vi "synchronize.vi"(8 "error in (no error)":errorcluster, 10 "input complex waveform":cluster{"t0":dbl, "dt":dbl, "Y":cdb[]}, 11 "Modulation Parameters In":T1={"RX Parameters"={"RX Oversample Factor"=4, "RX Sample Rate"=4000000.0, "Synchronization Options"={"Synchronization Method"=enum."Fixed Offset", "Symbol Timing Recovery Method "=enum."MT Allign To Ideal Symbols", "Fixed Offset"=0.0, "Frame Detection Method"=enum."", "Correct Frequency Offset"=FALSE}, "Channel Estimation/Equalization Parameters"={"Equalization Method"=enum."", "Channel Estimate Length"=0.0, "Equalizer Length"=0.0, "Equalizer Delay"=0.0}}, "TX/RX Shared Parameters"={"Modulation Type"=enum."OOK", "Packet Length"=128, "# of Iterations"=0.0, "Pulse Shaping Parameters"={"Pulse Shaping Filter"=enum."none", "Filter Length (symbols)"=32, "Filter Parameter"=0.8, "modulation type"=enum."FSK"}, "Header/Tail Control Information"={"Training Sequence Type"=enum."", "Zero Pad Length"=0.0}}}) -> (0 "error out":errorcluster, 2 "output complex waveform":cluster{"t0":dbl, "dt":dbl, "Y":cdb[]}, 3 "Modulation Parameters Out":T1={"RX Parameters"={"RX Oversample Factor"=4, "RX Sample Rate"=4000000.0, "Synchronization Options"={"Synchronization Method"=enum."Fixed Offset", "Symbol Timing Recovery Method "=enum."MT Allign To Ideal Symbols", "Fixed Offset"=0.0, "Frame Detection Method"=enum."", "Correct Frequency Offset"=FALSE}, "Channel Estimation/Equalization Parameters"={"Equalization Method"=enum."", "Channel Estimate Length"=0.0, "Equalizer Length"=0.0, "Equalizer Delay"=0.0}}, "TX/RX Shared Parameters"={"Modulation Type"=enum."OOK", "Packet Length"=128, "# of Iterations"=0.0, "Pulse Shaping Parameters"={"Pulse Shaping Filter"=enum."none", "Filter Length (symbols)"=32, "Filter Parameter"=0.8, "modulation type"=enum."FSK"}, "Header/Tail Control Information"={"Training Sequence Type"=enum."", "Zero Pad Length"=0.0}}})   [LabVIEW 2012]
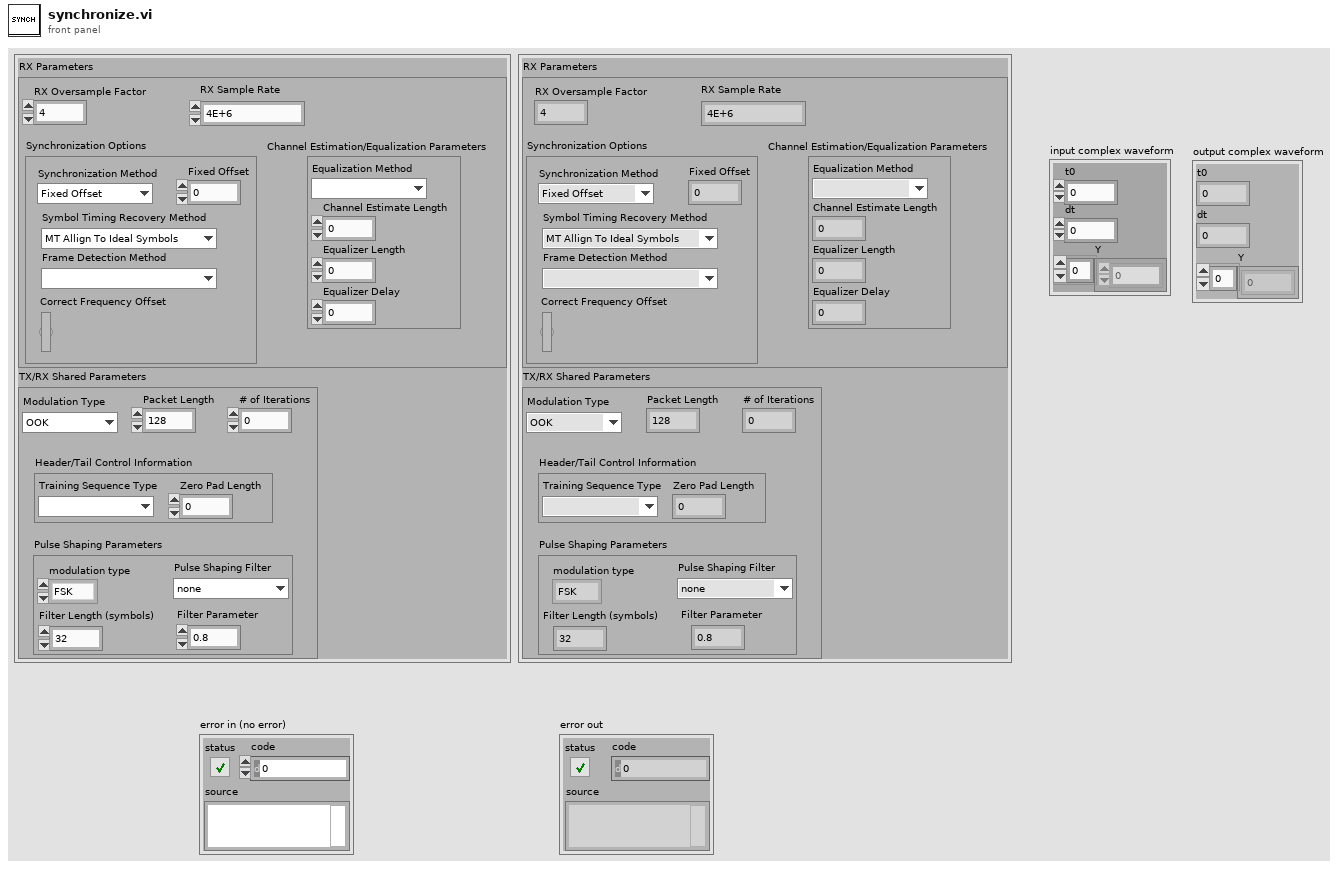
[diagram p1: front panel]
types:
  T1 = cluster{"RX Parameters":cluster{"RX Oversample Factor":i32, "RX Sample Rate":dbl, "Synchronization Options":cluster{"Synchronization Method":enum16{"Fixed Offset", "Timing Estimation", "Joint Timing and Channel Estimation"}, "Symbol Timing Recovery Method ":enum16{"MT Allign To Ideal Symbols", "Maximum Energy", "Early-Late Gate", "Gardner", "Fixed Offset"}, "Fixed Offset":dbl, "Frame Detection Method":enum16{""}, "Correct Frequency Offset":bool}, "Channel Estimation/Equalization Parameters":cluster{"Equalization Method":enum16{""}, "Channel Estimate Length":dbl, "Equalizer Length":dbl, "Equalizer Delay":dbl}}, "TX/RX Shared Parameters":cluster{"Modulation Type":enum16{"OOK", "FSK"}, "Packet Length":i32, "# of Iterations":dbl, "Pulse Shaping Parameters":cluster{"Pulse Shaping Filter":enum16{"none", "Raised Cosine", "Root Raised Cos", "Gaussian"}, "Filter Length (symbols)":i32, "Filter Parameter":dbl, "modulation type":enum16{"FSK", "PSK", "QAM", "MSK", "PAM", "ASK", "CPM"}}, "Header/Tail Control Information":cluster{"Training Sequence Type":enum16{""}, "Zero Pad Length":dbl}}}
  T2 = enum16{"Fixed Offset", "Timing Estimation", "Joint Timing and Channel Estimation"}
  T3 = cluster{"RX Parameters":cluster{"RX Oversample Factor":i32, "RX Sample Rate":dbl, "Synchronization Options":cluster{"Synchronization Method":enum16{"Fixed Offset", "Timing Estimation", "Joint Timing and Channel Estimation"}, "Symbol Timing Recovery Method ":enum16{"MT Allign To Ideal Symbols", "Maximum Energy", "Early-Late Gate", "Gardner", "Fixed Offset"}, "Fixed Offset":i32, "Frame Detection Method":enum16{""}, "Correct Frequency Offset":bool}, "Channel Estimation/Equalization Parameters":cluster{"Equalization Method":enum16{""}, "Channel Estimate Length":dbl, "Equalizer Length":dbl, "Equalizer Delay":dbl}}, "TX/RX Shared Parameters":cluster{"Modulation Type":enum16{"OOK", "FSK"}, "Packet Length":i32, "# of Iterations":dbl, "Pulse Shaping Parameters":cluster{"Pulse Shaping Filter":enum16{"none", "Raised Cosine", "Root Raised Cos", "Gaussian"}, "Filter Length (symbols)":i32, "Filter Parameter":dbl, "modulation type":enum16{"FSK", "PSK", "QAM", "MSK", "PAM", "ASK", "CPM"}}, "Header/Tail Control Information":cluster{"Training Sequence Type":enum16{""}, "Zero Pad Length":dbl}}}
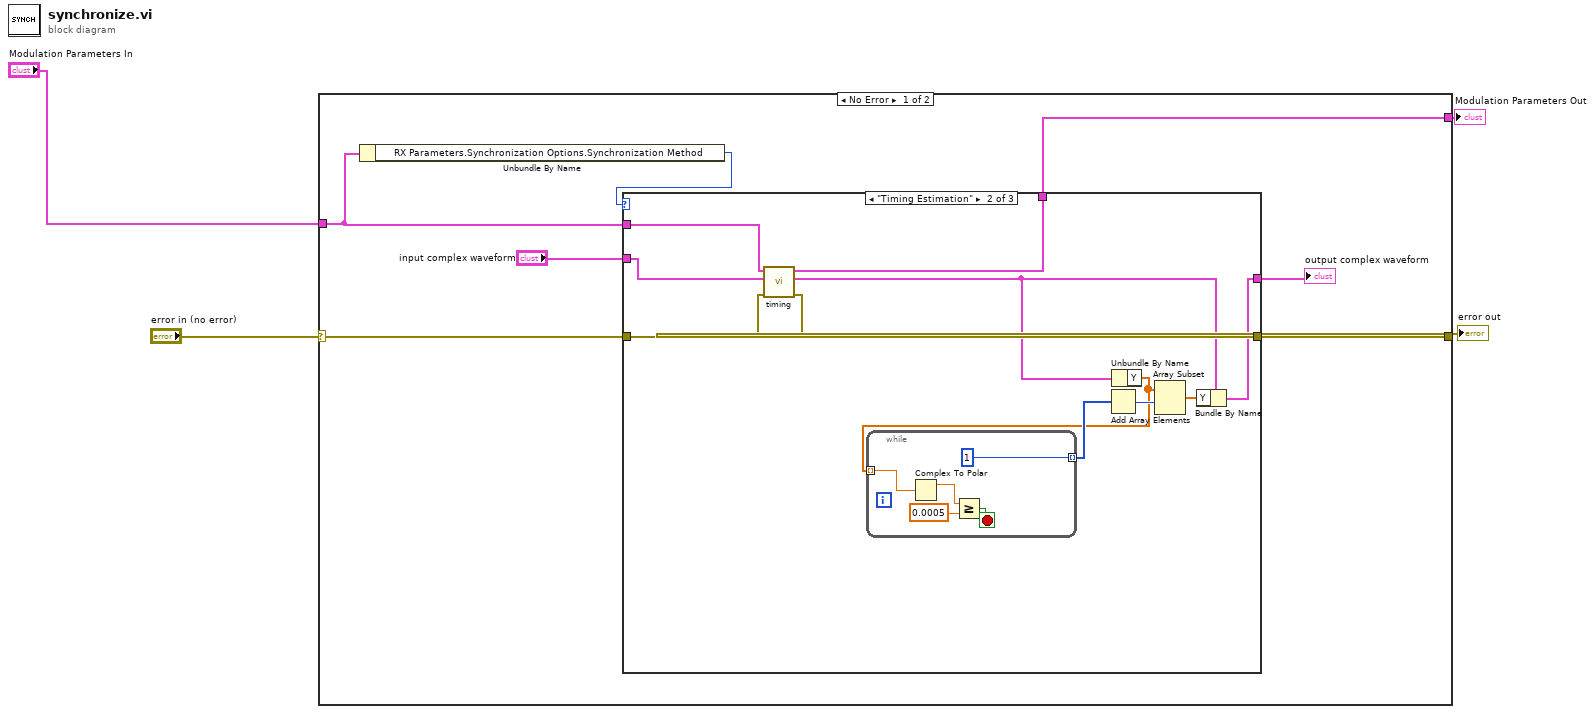
[diagram p0: block diagram]
diagram:
  n1 = case shown="No Error" "error in (no error)" {
    selector: "error in (no error)" -> [w8 w35]
    tunnel: [w7 w35] -> w3
    tunnel: "Modulation Parameters In" -> [w9 w34]
    tunnel: [w6 w34] -> w1
    frame No Error {
      n2 = Unbundle By Name(w9) -> ("RX Parameters.Synchronization Options.Synchronization Method"=w11:T2)
      n3 = case shown="\"Timing Estimation\"" w11 {
        tunnel: "input complex waveform" -> [w13 w24 w32]
        tunnel: w9 -> [w14 w25 w33]
        tunnel: w8 -> [w12 w23 w31]
        tunnel: [w12 w22 w31] -> w7
        tunnel: [w14 w21 w33] -> w6
        tunnel: [w13 w17 w32] -> w5
        frame "Fixed Offset", Default {
          # "To be implemented"
        }
        frame "Timing Estimation" {
          n4 = call "timing.vi"("error in (no error)"=w23, "input complex waveform"=w24, "Modulation Parameters In"=w25) -> ("error out"=w22:errorcluster, "output complex waveform"=w18:cluster{"t0":dbl, "dt":dbl, "Y":cdb[]}, "Modulation Parameters Out"=w21:T3)  [unwired: 5 in, 1 out]
          n5 = Unbundle By Name(w18) -> ("Y"=w16:cdb[])
          n6 = while {
            tunnel: w16 -> [w29] mode=indexing
            tunnel: [1] -> w20 mode=indexing
            stop <- w27 stop-if-true
            n7 = Complex To Polar(r * e^(i*theta)=w29) -> (r=w30:dbl)  [unwired: 1 out]
            n8 = Greater Or Equal?(x=w30, y=0.0005) -> (x >= y?=w27:bool)
          }
          n9 = Add Array Elements(numeric array=w20) -> (sum=w19:i32)
          n10 = Array Subset(array=w16, index=w19) -> (w15:cdb[])  [unwired: 1 in]
          n11 = Bundle By Name(cluster=w18, "Y"=w15) -> (w17:cluster{"t0":dbl, "dt":dbl, "Y":cdb[]})
        }
        frame "Joint Timing and Channel Estimation" {
          # "To be implemented"
        }
      }
      "output complex waveform" <- w5
    }
    frame Error {
    }
  }
  "error out" <- w3
  "Modulation Parameters Out" <- w1
